vi "Do.vi"(8 "error in (no error)":errorcluster, 10 "Steps":i32, 11 "Proto In":refnum<class "Proto.lvclass">) -> (0 "error out":errorcluster, 2 "Possible Coords":cluster{"Row":i32, "Col":i32}[](array[cluster]), 3 "Proto Out":refnum<class "Proto.lvclass">)   [LabVIEW 2021, in "Proto.lvclass"]
uses:
  Proto.lvclass
  Proto.lvclass/Proto.ctl
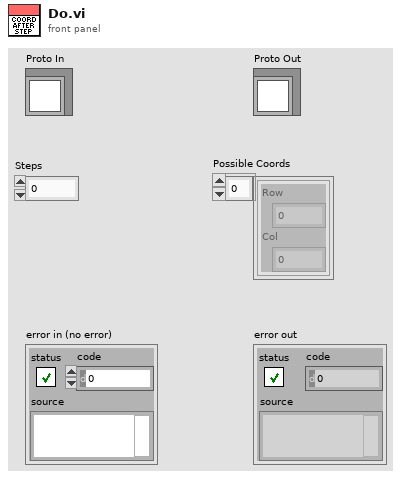
[diagram p1: front panel]
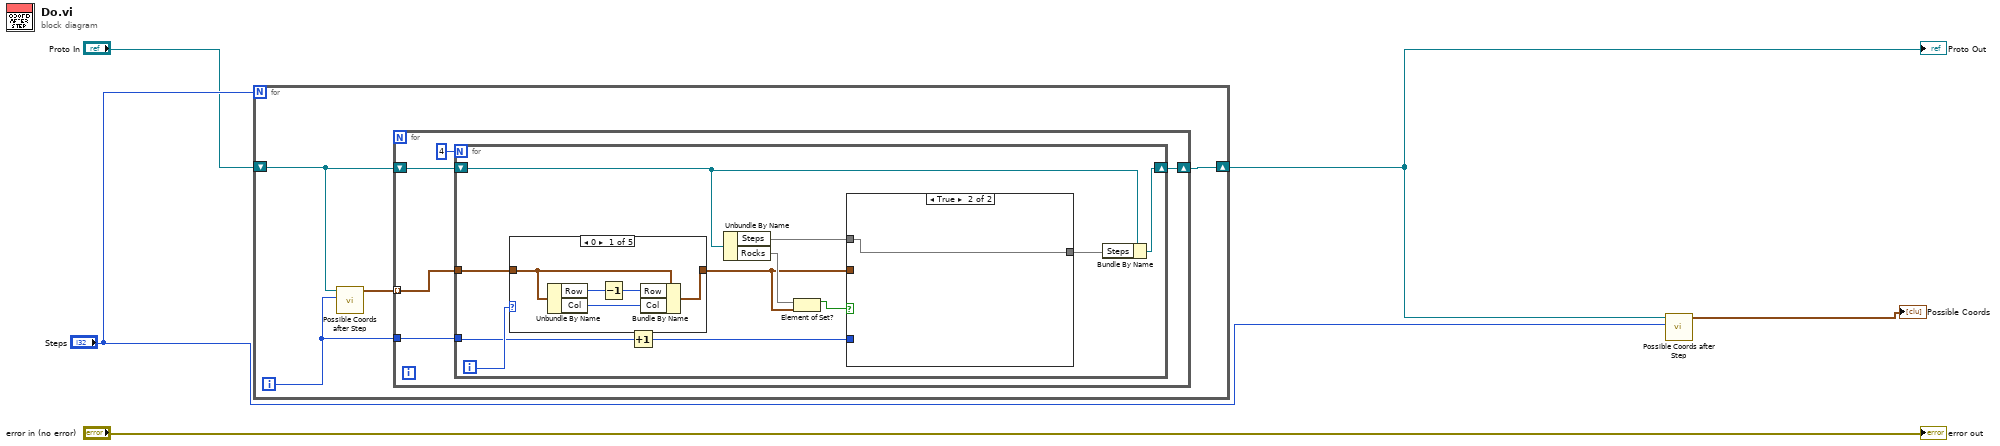
[diagram p0: block diagram]
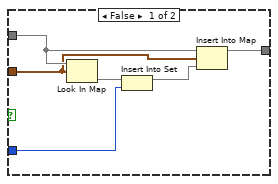
[diagram p2: hidden frame]
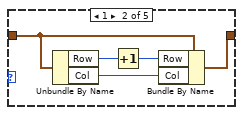
[diagram p3: hidden frame]
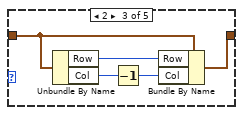
[diagram p4: hidden frame]
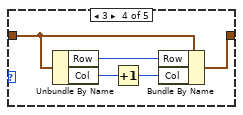
[diagram p5: hidden frame]
diagram:
  n1 = for {
    N: "Steps" -> [_]
    shift-right: [w7] -> w1
    shift-left: "Proto In" -> [w8]
    i -> [w6]
    n2 = call "Possible Coords after Step.vi"("Steps"=w6, "Proto in"=w8) -> ("Array"=w9:cluster{"Row":i32, "Col":i32}[])  [unwired: 9 in]
    n3 = for {
      tunnel: w9 -> [w12] mode=indexing
      shift-right: [w13] -> w7
      shift-left: w8 -> [w14]
      tunnel: w6 -> [w10]
      n4 = for {
        N: 4 -> [_]
        shift-right: [w23] -> w13
        shift-left: w14 -> [w25]
        tunnel: w12 -> [w21]
        tunnel: w10 -> [w19]
        i -> [w20]
        n5 = case shown="0" w20 {
          tunnel: w21 -> [w37 w42 w47 w52 w53]
          tunnel: [w36 w41 w46 w51 w53] -> w16
          frame 0 {
            n6 = Unbundle By Name(w37) -> ("Row"=w35:i32, "Col"=w34:i32)
            n7 = Decrement(x=w35) -> (x-1=w33:i32)
            n8 = Bundle By Name(cluster=w37, "Row"=w33, "Col"=w34) -> (w36:cluster{"Row":i32, "Col":i32})
          }
          frame 1 {
            n9 = Unbundle By Name(w42) -> ("Row"=w40:i32, "Col"=w39:i32)
            n10 = Increment(x=w40) -> (x+1=w38:i32)
            n11 = Bundle By Name(cluster=w42, "Row"=w38, "Col"=w39) -> (w41:cluster{"Row":i32, "Col":i32})
          }
          frame 2 {
            n12 = Unbundle By Name(w47) -> ("Row"=w45:i32, "Col"=w44:i32)
            n13 = Decrement(x=w44) -> (x-1=w43:i32)
            n14 = Bundle By Name(cluster=w47, "Row"=w45, "Col"=w43) -> (w46:cluster{"Row":i32, "Col":i32})
          }
          frame 3 {
            n15 = Unbundle By Name(w52) -> ("Row"=w50:i32, "Col"=w49:i32)
            n16 = Increment(x=w49) -> (x+1=w48:i32)
            n17 = Bundle By Name(cluster=w52, "Row"=w50, "Col"=w48) -> (w51:cluster{"Row":i32, "Col":i32})
          }
          frame Default {
          }
        }
        n18 = Increment(x=w19) -> (x+1=w18:i32)
        n19 = Unbundle By Name(w25) -> ("Steps"=w22:map{cluster{"Row":i32, "Col":i32}, set{i32}}, "Rocks"=w17:set{cluster{"Row":i32, "Col":i32}})
        n20 = Element of Set?(10:w16, 11:w17) -> (3:w15:bool)
        n21 = case shown="True" w15 {
          tunnel: [w31 w32] -> w24
          tunnel: w22 -> [w30 w32]
          tunnel: w18 -> [w27 _]
          tunnel: w16 -> [w26 _]
          frame False {
            n22 = Look In Map(map=w30, key=w26) -> (value=w29:set{i32})  [unwired: 1 in, 1 out]
            n23 = Insert Into Set(10:w27, 11:w29) -> (3:w28:set{i32})  [unwired: 1 out]
            n24 = Insert Into Map(map in=w30, key=w26, value=w28) -> (map out=w31:map{cluster{"Row":i32, "Col":i32}, set{i32}})  [unwired: 2 out]
          }
          frame True {
          }
        }
        n25 = Bundle By Name(cluster=w25, "Steps"=w24) -> (w23:refnum<class "Proto.lvclass">)
      }
    }
  }
  "Proto Out" <- w1
  n26 = call "Possible Coords after Step.vi"("Steps"="Steps", "Proto in"=w1) -> ("Array"=→"Possible Coords":cluster{"Row":i32, "Col":i32}[])  [unwired: 9 in]
  "error out" <- "error in (no error)"
